vi "motor_move_event.vi"() -> ()   [LabVIEW 2013]
panel:
  out "motor status event":refnum<user-event>
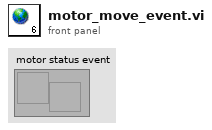
[diagram p1: front panel]
diagram:
